vi "Pre Launch Init.vi"(11 "DAQ Device in":refnum<class "DAQ Device.lvclass">) -> (0 "error out":errorcluster, 3 "DAQ Device out":refnum<class "DAQ Device.lvclass">)   [LabVIEW 2014, in "DAQ Device.lvclass"]
doc: "(<B>Filename</B>: Actor Framework.lvlib:Actor.lvclass:Pre Launch Init.vi)\n\nDefines behavior that occurs after the Launch Actor method is invoked but before the actor's Actor Core method begins running.\n\nThe Pre Launch Init method is guaranteed to finish before the Launch Actor method returns to its caller and before the actor itself receives any messages. Any references that the Pre Launch Init method obtains are guaranteed to have the same lifetime as the actor itself. Any errors that the Pre Launch Init method returns will abort the launch.\n\nBy default, this method does nothing. A descendant class may override it to define behavior."
uses:
  DAQ Device.lvclass
  DAQ Device.lvclass/DAQ Device.ctl
  Session APIs/Session Log/System Log.lvclass
  <userlib>/_Session Fwk/Session - Root.lvclass
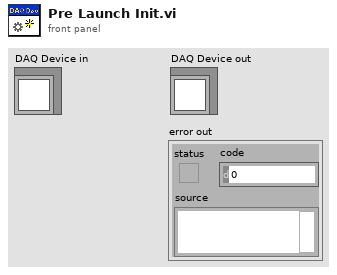
[diagram p1: front panel]
types:
  T1 = typedef "Session - Root.lvclass/Session Handle.ctl" = refnum<data-value>
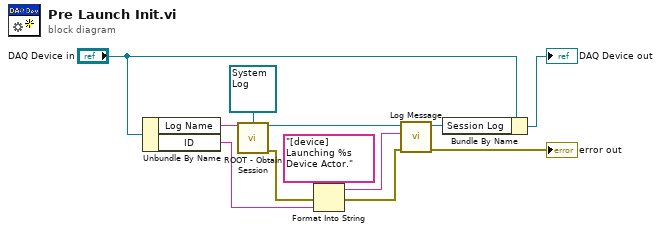
[diagram p0: block diagram]
diagram:
  n1 = Unbundle By Name("DAQ Device in") -> ("Log Name"=w12:string, "ID"=w2:string)
  n2 = call <userlib>:"ROOT - Obtain Session.vi"("Session Name ()"=w12, "OBJ - Session"=refnum<class "System Log.lvclass"> refnum ("Sys Log")) -> ("Session Handle"=w8:T1, "error out"=w5:errorcluster)  [unwired: 11 in, 1 out]
  n3 = Format Into String(format string="[device] Launching %s Device Actor.", error in=w5, w2) -> (resulting string=w1:string, error out=w4:errorcluster)  [unwired: 1 in]
  n4 = call "Log Message.vi"("error in"=w4, "MSG In"=w1, "session in"=w8) -> ("error out"=→"error out":errorcluster, "session out"=w6:T1)  [unwired: 7 in]
  n5 = Bundle By Name(cluster="DAQ Device in", "Session Log"=w6) -> (→"DAQ Device out":refnum<class "DAQ Device.lvclass">)
